vi "Subtract.vi"(10 "x":dbl, 11 "y":dbl) -> (2 "x-y":dbl)   [LabVIEW 2021]
panel:
  in  "Boolean":bool
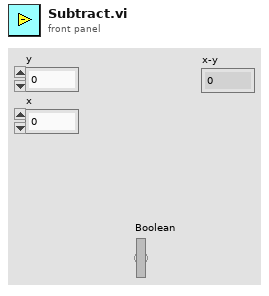
[diagram p1: front panel]
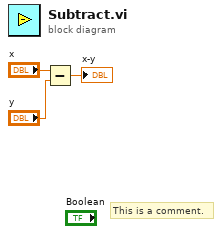
[diagram p0: block diagram]
diagram:
  # "This is a comment."
  n1 = Subtract(x="x", y="y") -> (x-y=→"x-y":dbl)
